vi "Configure Setpoint Ramp Rate.vi"(8 "error in (no error)":errorcluster, 9 "Ramp Rate (9999)":dbl=9999.0 min=0.0 max=9999.0 step=1.0, 11 "VISA resource name":refnum<visa-resource-name>) -> (0 "error out":errorcluster, 3 "VISA resource name out":refnum<visa-resource-name>)   [LabVIEW 2012, in "Temptronic TP04300.lvlib"]
doc: "This VI configures the setpoint's ramp rate.\n\n<b>Setpoint ramp rate</b>\n\nValid Range: 0 to 9999.0\nDefault Value: 9999.0"
uses:
  <instrlib>/Temptronic TP04300/Temptronic TP04300.lvlib
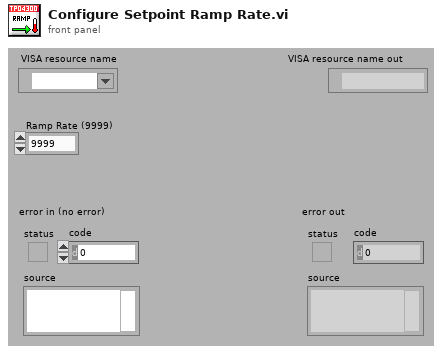
[diagram p1: front panel]
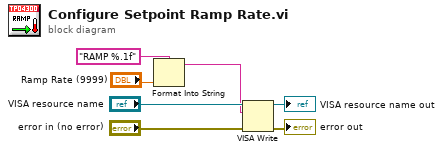
[diagram p0: block diagram]
diagram:
  n1 = Format Into String(format string="RAMP %.1f" ("multi-line string"), "Ramp Rate (9999)") -> (resulting string=w3:string)  [unwired: 2 in, 1 out]
  n2 = VISA Write(VISA resource name="VISA resource name", write buffer=w3, error in (no error)="error in (no error)") -> (VISA resource name out=→"VISA resource name out":refnum<visa-resource-name>, error out=→"error out":errorcluster)  [unwired: 1 out]
